vi "GetSettingGeneral.vi"(8 "error in (no error)":errorcluster, 11 "Gviewer in":refnum<class "Gviewer.lvclass">) -> (0 "error out":errorcluster, 3 "Gviewer out":refnum<class "Gviewer.lvclass">)   [LabVIEW 2020, in "Sgraph_lib_V1.lvlib" / "Gviewer.lvclass"]
doc: "Get General Settings\n(applicable for all instances of Gviewer simultaneously)"
uses:
  Gviewer.lvclass
  controls/SettingsGeneral.ctl
  Gviewer.lvclass/Gviewer.ctl
panel:
  out "SettingsGeneral":T1
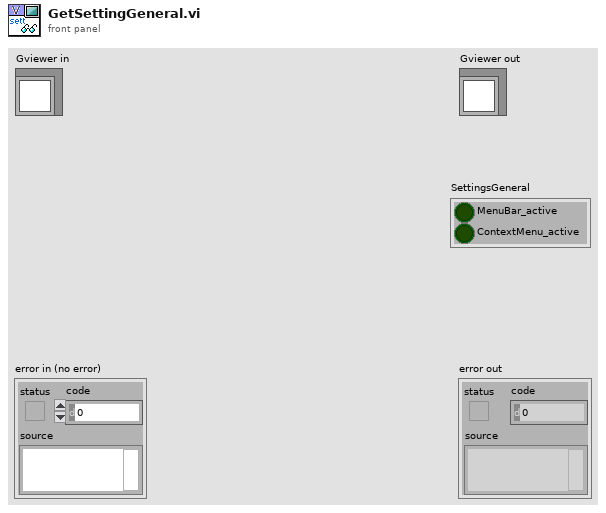
[diagram p1: front panel]
types:
  T1 = typedef "Sgraph_lib_V1.lvlib/Gviewer.lvclass/SettingsGeneral.ctl" = cluster{"MenuBar_active":bool, "ContextMenu_active":bool}
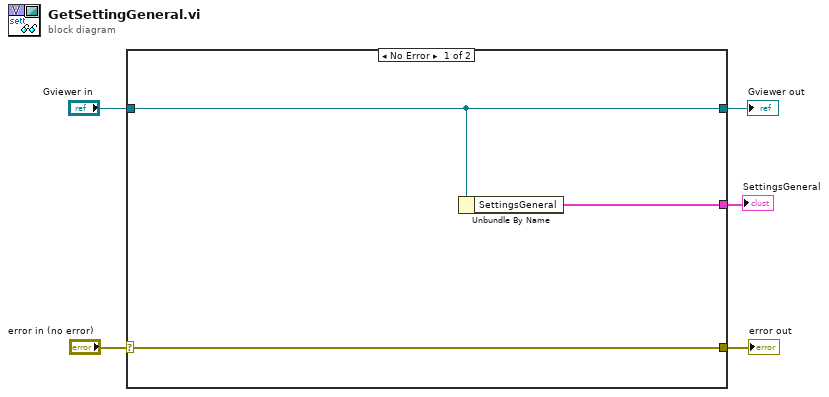
[diagram p0: block diagram]
diagram:
  n1 = case shown="No Error" "error in (no error)" {
    selector: "error in (no error)" -> [w8 w10]
    tunnel: [w8 w10] -> w4
    tunnel: [w7 w9] -> w2
    tunnel: "Gviewer in" -> [w7 w9]
    tunnel: [w6 _] -> w1
    frame No Error {
      n2 = Unbundle By Name(w7) -> ("SettingsGeneral"=w6:T1)
    }
    frame Error {
    }
  }
  "error out" <- w4
  "Gviewer out" <- w2
  "SettingsGeneral" <- w1
